vi "XYZStage-Read position command.vi"(8 "error in (no error)":errorcluster, 9 "Z Stage":T1, 10 "XY Stage config cluster":T2, 11 "UI ctrl refs":T3) -> (0 "error out":errorcluster, 2 "Coordinates":cluster{"X":sgl, "Y":sgl, "Z":sgl})   [LabVIEW 2020]
doc: "Reads the XYZ Stage coordinates"
uses:
  Typedefs/UI ctrl refs cluster.ctl
  Typedefs/Laser control knob.ctl
  Typedefs/Frame Size.ctl
  Typedefs/Plane Mode.ctl
  Typedefs/PMT control knob.ctl
  Typedefs/XY Stage_Move.ctl
  Typedefs/test_fpga_control.ctl
  Acquisition/Typedefs/Ref DAQ Param.ctl
  User Interface/Misc/Experiment Type.ctl
  User Interface/Misc/Biology Information.ctl
  Typedefs/XY Stage config cluster.ctl
  Typedefs/Z Stage config cluster.ctl
  Global Variables/General Globals.vi
  <userlib>/_MGI/Application Control/MGI Change Detector/MGI Change Detector (T).vi
panel:
  out "number":dbl format="%#.3f"
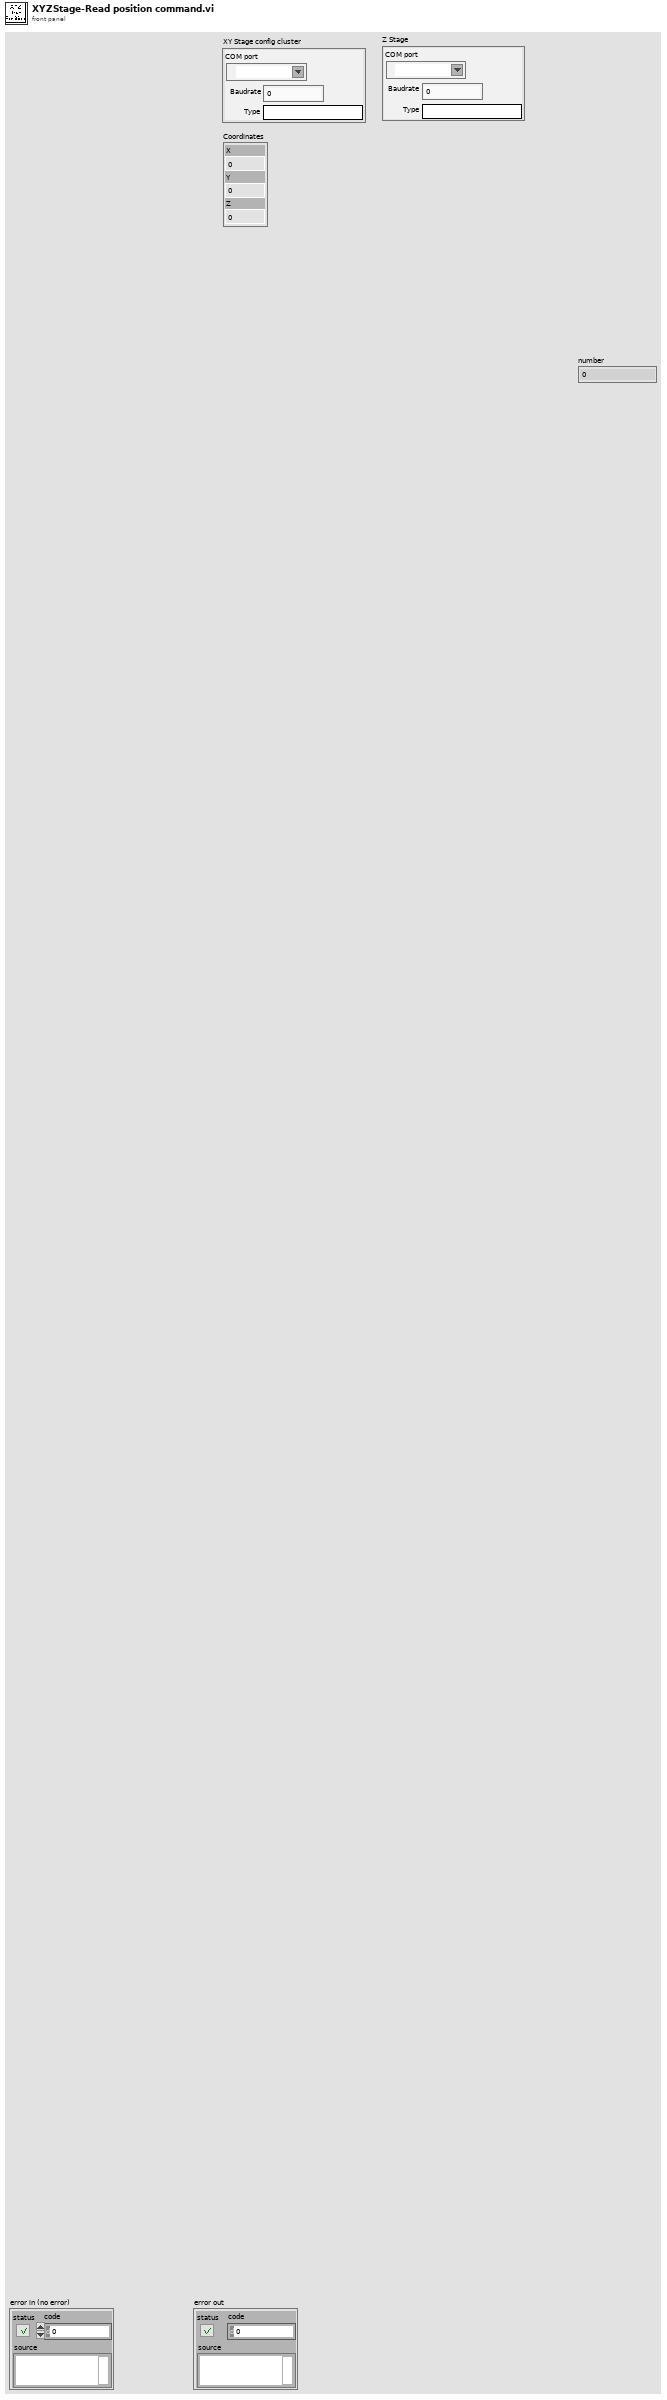
[diagram p1: front panel]
types:
  T1 = typedef "Z Stage config cluster.ctl" = cluster{"COM port":refnum<visa-resource-name>, "Baudrate":i32, "Type":string}
  T2 = typedef "XY Stage config cluster.ctl" = cluster{"COM port":refnum<visa-resource-name>, "Baudrate":i32, "Type":string}
  T3 = typedef "UI ctrl refs cluster.ctl" = cluster{"Top level VI path":path, "Top level VI ref":refnum<vi>, "User menu ref":refnum<k9>, "Sub Panel control":refnum<vi>, "Imaging Param Tab":refnum<vi>, "Occurrence-Start drivers":refnum<k4>, "Occurrence-Speed logging initialised":refnum<k4>, "Occurrence-XYZ stage initialised":refnum<k4>, "Exit button":refnum<vi>, "Status ind":refnum<vi>, "Set as origin":refnum<vi>, "Speed Logging":refnum<vi>, "Time Lapse":refnum<vi>, "Live Imaging":refnum<vi>, "AOL Z Stack":refnum<vi>, "Motor Z Stack":refnum<vi>, "Funct Acq button":refnum<vi>, "Hard Shutter":refnum<vi>, "Virtual Shutter":refnum<vi>, "Laser Power":refnum<vi>, "AOL Mode":refnum<vi>, "Frame Size":refnum<vi>, "Field of View":refnum<vi>, "Dwell Time":refnum<vi>, "Zoom":refnum<vi>, "AOL Z":refnum<vi>, "Objective":refnum<vi>, "Axis":refnum<vi>, "Paths & Names":refnum<vi>, "Experiment folder path (ind.)":refnum<vi>, "Last State (Ind.)":refnum<vi>, "Averages":refnum<vi>, "Angle (degrees)":refnum<vi>, "X centre":refnum<vi>, "Y centre":refnum<vi>, "Plane Mode":refnum<vi>, "# Planes":refnum<vi>, "Z Start":refnum<vi>, "Z Stop":refnum<vi>, "Z Step":refnum<vi>, "PMT 1":refnum<vi>, "PMT 2":refnum<vi>, "Stage XYZ Position":refnum<vi>, "Pockels@Z Start":refnum<vi>, "Pockels@Z Stop":refnum<vi>, "Obtain Z Start":refnum<vi>, "Obtain Z Stop":refnum<vi>, "Live stim.trig.period":refnum<vi>, "Live stim.trig.enable":refnum<vi>, "Movement Correction":refnum<vi>, "Load Reference Image":refnum<vi>, "XY Stage Move":refnum<vi>, "MovCor Cluster":refnum<vi>, "RefDAQParam":refnum<vi>, "Funct. Acq. Pockels Modulation":refnum<vi>, "Ref Laser Power":refnum<vi>, "Enable Video Recording":refnum<vi>, "Video Record-Live Imaging":refnum<vi>, "Video Record-Funct acq":refnum<vi>, "Reference Source":refnum<vi>, "AOL Z-stack Chirps Ready (ind)":refnum<vi>, "Target time between mov.cor. ref triggers (ms)":refnum<vi>, "Funct. Acq. Ref frame save":refnum<vi>, "Tracking button":refnum<vi>, "Show ref plots window":refnum<vi>, "Center freq ind (nm)":refnum<vi>, "Pickup mode (ind)":refnum<vi>, "Logging queue (ind)":refnum<vi>, "Back aperture power (ind.)":refnum<vi>, "Power after objective (ind.)":refnum<vi>, "Switch user":refnum<vi>, "Ls1 Conn. Status":refnum<vi>, "Ls1Tuning Status":refnum<vi>, "Ls1 Faults":refnum<vi>, "Ls1 Connection":refnum<vi>, "Ls1 Mode":refnum<vi>, "Ls1 POWER [mW]":refnum<vi>, "Ls1Shutter":refnum<vi>, "Ls1 Wavelength":refnum<vi>, "Ls1 Note":refnum<vi>, "Ls1 Confirm Wav":refnum<vi>, "Ls1 PreChrp Prism1":refnum<vi>, "Ls1 PreChrp Prism2":refnum<vi>, "Ls1 wav top Ind":refnum<vi>, "Ls1 power top Ind":refnum<vi>, "Ls1 Pump peak Hold":refnum<vi>, "Ls1 Status Ind":refnum<vi>, "Ls1 wav cancel":refnum<vi>, "Experiment Type":refnum<vi>, "Biology Information":refnum<vi>, "Camera recording status":refnum<vi>, "Optimise Obj. Pos.":refnum<vi>}
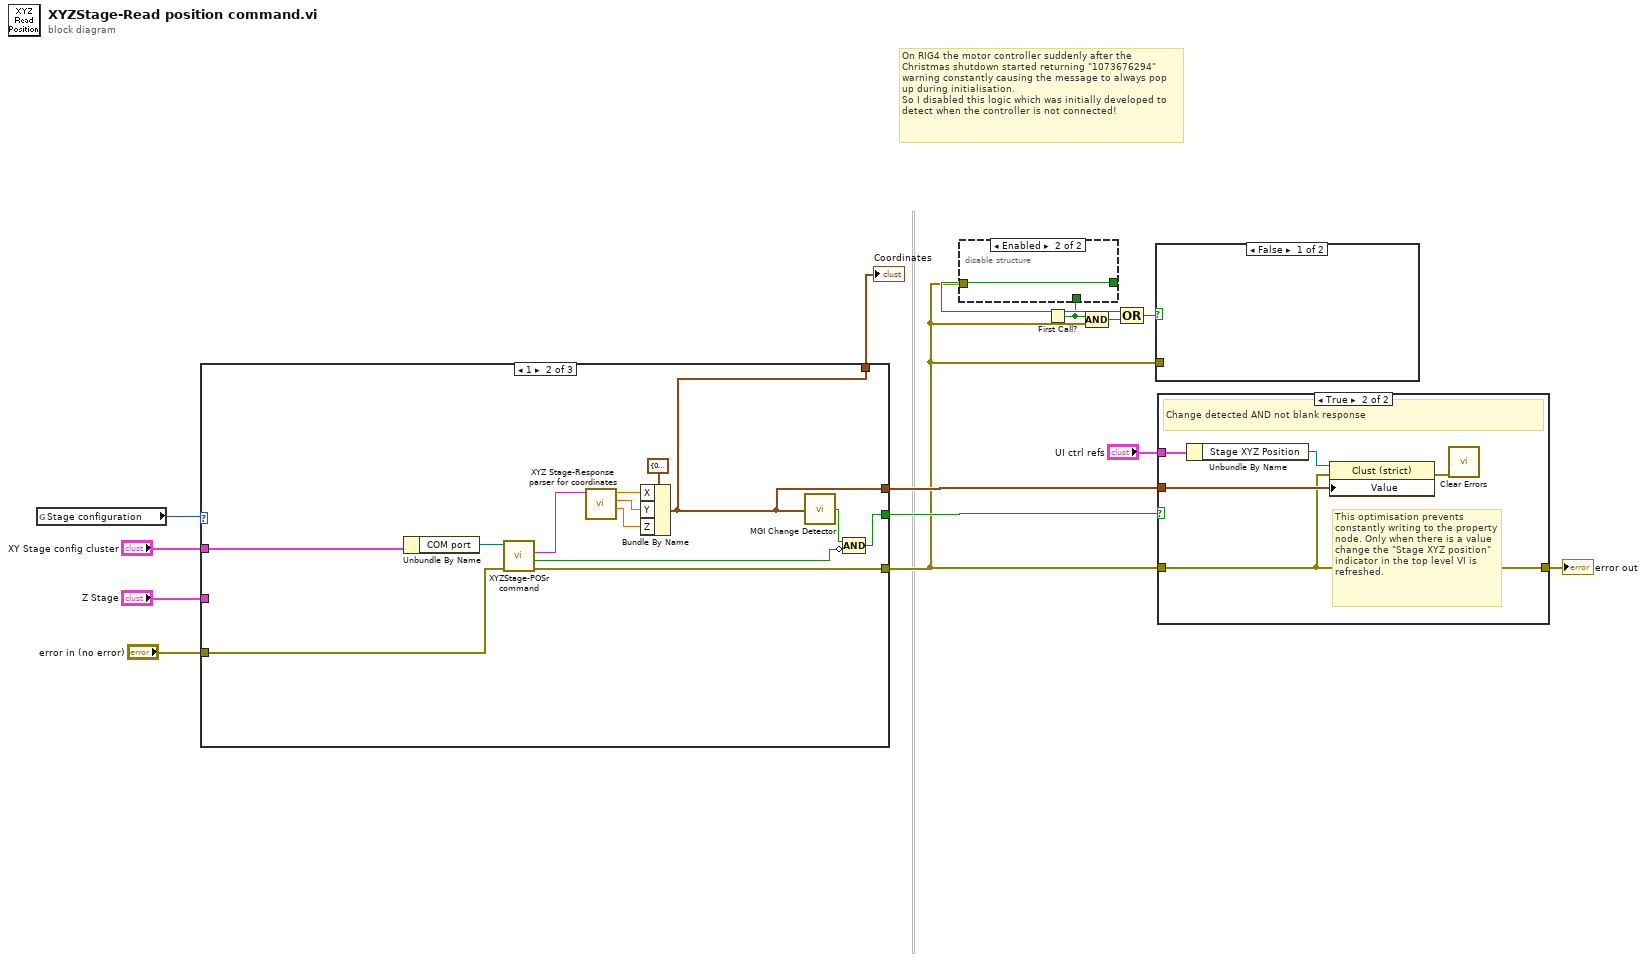
[diagram p0: block diagram]
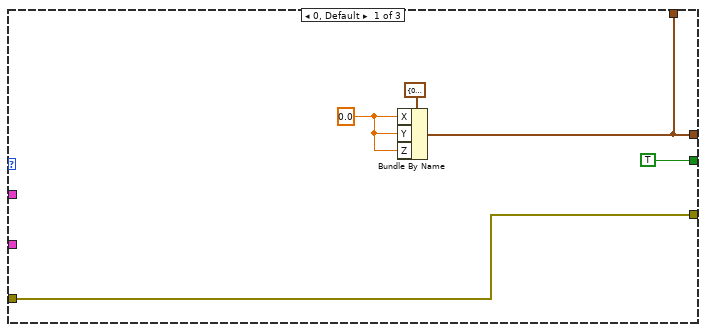
[diagram p2: hidden frame]
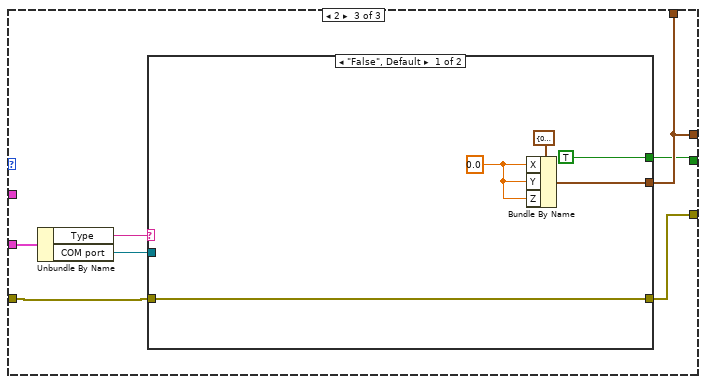
[diagram p3: hidden frame]
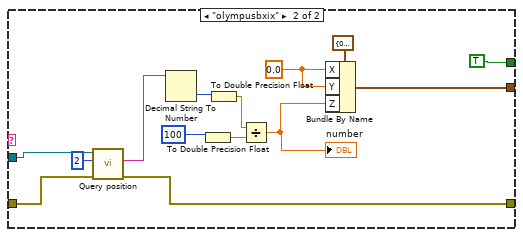
[diagram p4: hidden frame]
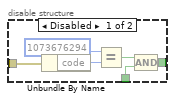
[diagram p5: hidden frame]
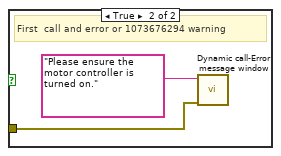
[diagram p6: hidden frame]
diagram:
  # "On RIG4 the motor controller suddenly after the Christmas shutdown started returning \"1073676294\" warning constantly causing the message to always pop up during initialisation.\nSo I disabled this logic which was initially developed to detect when the controller is not connected!"
  n1 = global read "General Globals.vi" "Stage configuration"() -> (w3:i32)
  n2 = case shown="1" w3 {
    tunnel: [w16 w20 w35] -> w12
    tunnel: [TRUE w24 w34] -> w11
    tunnel: [w18 w23 w33] -> w6
    tunnel: "error in (no error)" -> [w18 w22 w36]
    tunnel: "XY Stage config cluster" -> [_ w21 _]
    tunnel: [w16 w20 w35] -> w2
    tunnel: "Z Stage" -> [_ _ w39]
    frame 0, Default {
      w17 = sgl 0.0 ("X")
      n3 = Bundle By Name(cluster=cluster{"X":sgl, "Y":sgl, "Z":sgl} {"X"=0.0, "Y"=0.0, "Z"=0.0} ("Stage XYZ Position"), "X"=w17, "Y"=w17, "Z"=w17) -> (w16:cluster{"X":sgl, "Y":sgl, "Z":sgl})
    }
    frame 1 {
      n4 = Unbundle By Name(w21) -> ("COM port"=w28:refnum<visa-resource-name>)
      n5 = call "XYZStage-POSr command.vi"("Error in"=w22, "VISA Refnum in"=w28) -> ("Error out"=w23:errorcluster, "Empty response string"=w25:bool, "read string"=w27:string)  [unwired: 6 in, 1 out]
      n6 = call "XYZ Stage-Response parser for coordinates.vi"("Filtered response string (no CR)"=w27) -> ("Z"=w32:sgl, "Y"=w31:sgl, "X"=w30:sgl)  [unwired: 7 in, 1 out]
      n7 = Bundle By Name(cluster=cluster{"X":sgl, "Y":sgl, "Z":sgl} {"X"=0.0, "Y"=0.0, "Z"=0.0} ("Stage XYZ Position"), "X"=w30, "Y"=w31, "Z"=w32) -> (w20:cluster{"X":sgl, "Y":sgl, "Z":sgl})
      n8 = call-poly <userlib>:"MGI Change Detector.vi"("Value"=w20) -> ("Changed?"=w26:bool)
      n9 = Compound Arithmetic op=AND(w26, invert w25) -> (w24:bool)
    }
    frame 2 {
      n10 = Unbundle By Name(w39) -> ("Type"=w38:string, "COM port"=w37:refnum<visa-resource-name>)
      n11 = case shown="\"False\", Default" w38 {
        tunnel: w37 -> [_ w53]
        tunnel: w36 -> [w40 w52]
        tunnel: [w42 w47] -> w35
        tunnel: [TRUE TRUE] -> w34
        tunnel: [w40 w45] -> w33
        frame "False", Default {
          w43 = sgl 0.0 ("X")
          n12 = Bundle By Name(cluster=cluster{"X":sgl, "Y":sgl, "Z":sgl} {"X"=0.0, "Y"=0.0, "Z"=0.0} ("Stage XYZ Position"), "X"=w43, "Y"=w43, "Z"=w43) -> (w42:cluster{"X":sgl, "Y":sgl, "Z":sgl})
        }
        frame "olympusbxix" {
          w49 = sgl 0.0 ("X")
          n13 = call "Query position.vi"("error in (no error)"=w52, "Device Number (1)"=2, "VISA Resource Name"=w53) -> ("error out"=w45:errorcluster, "Result"=w58:string)  [unwired: 6 in, 1 out]
          n14 = Decimal String To Number(string=w58) -> (number=w57:i32)  [unwired: 2 in, 1 out]
          n15 = To Double Precision Float(number=100 ("y")) -> (double precision float=w56:dbl)
          n16 = To Double Precision Float(number=w57) -> (double precision float=w54:dbl)
          n17 = Divide(x=w54, y=w56) -> (x/y=w48:dbl)
          "number" <- w48
          n18 = Bundle By Name(cluster=cluster{"X":sgl, "Y":sgl, "Z":sgl} {"X"=0.0, "Y"=0.0, "Z"=0.0} ("Stage XYZ Position"), "X"=w49, "Y"=w49, "Z"=w48) -> (w47:cluster{"X":sgl, "Y":sgl, "Z":sgl})
        }
      }
    }
  }
  "Coordinates" <- w2
  n19 = First Call?() -> (First Call?: T/F=w9:bool)
  n20 = disable-structure shown="Enabled" {
    disable-tunnel: [w61 _] -> w10
    disable-tunnel: w9 -> [w60 _]
    disable-tunnel: w6 -> [w59 _]
    frame Disabled {
      n21 = Unbundle By Name(w59) -> ("code"=w64:i32)
      n22 = Equal?(x=1073676294, y=w64) -> (x = y?=w62:bool)
      n23 = Compound Arithmetic op=AND(w62, w60) -> (w61:bool)
    }
    frame Enabled {
    }
  }
  n24 = Compound Arithmetic op=AND(w9, w6) -> (w8:bool)
  n25 = Compound Arithmetic op=OR(w10, w8) -> (w7:bool)
  n26 = case shown="False" w7 {
    tunnel: w6 -> [_ w65]
    frame False {
    }
    frame True {
      # "First  call and error or 1073676294 warning"
      n27 = call "Dynamic call-Error message window.vi"("error in (no error)"=w65, "Error Message"="Please ensure the motor controller is turned on.") -> ()  [unwired: 9 in, 1 out]
    }
  }
  n28 = case shown="True" w11 {
    tunnel: [w67 w68] -> w14
    tunnel: w6 -> [w67 w68]
    tunnel: w12 -> [_ w72]
    tunnel: "UI ctrl refs" -> [_ w71]
    frame False {
      # "No change OR blank response"
    }
    frame True {
      # "This optimisation prevents constantly writing to the property node. Only when there is a value change the \"Stage XYZ position\" indicator in the top level VI is refreshed."
      # "Change detected AND not blank response"
      n29 = Unbundle By Name(w71) -> ("Stage XYZ Position"=w70:refnum<vi>)
      n30 = property on="Property Node" class="Clust (strict)"(reference=w70, error in=w68, "Value"=w72) -> (error out=w69:errorcluster)  [unwired: 1 out]
      n31 = call <vilib>:"Clear Errors.vi"("error in (no error)"=w69) -> ()  [unwired: 5 in, 2 out]
    }
  }
  "error out" <- w14
